vi "Read userEventRef.vi"(8 "error in (no error)":errorcluster, 11 "BoolUserEventStopMechanism In":refnum<class "BoolUETaskChannel.lvclass">) -> (0 "error out":errorcluster, 2 "stopUserEvent":refnum<user-event>, 3 "BoolUserEventStopMechanism Out":refnum<class "BoolUETaskChannel.lvclass">)   [LabVIEW 2023, in "TLC_Daemon.lvlib" / "BoolUETaskChannel.lvclass"]
uses:
  BoolUETaskChannel.lvclass
  BoolUETaskChannel.lvclass/BoolUETaskChannel.ctl
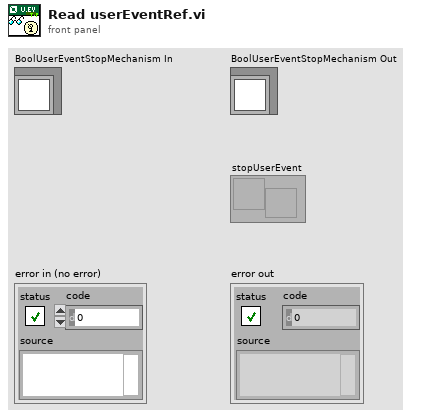
[diagram p1: front panel]
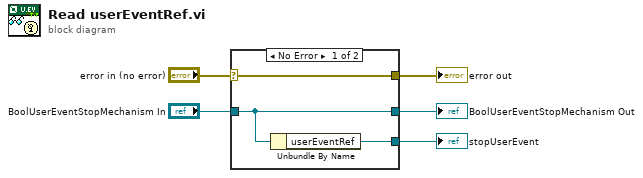
[diagram p0: block diagram]
diagram:
  n1 = case shown="No Error" "error in (no error)" {
    selector: "error in (no error)" -> [w8 w9]
    tunnel: [w8 w9] -> w4
    tunnel: [w7 w10] -> w2
    tunnel: "BoolUserEventStopMechanism In" -> [w7 w10]
    tunnel: [w6 _] -> w1
    frame No Error {
      n2 = Unbundle By Name(w7) -> ("userEventRef"=w6:refnum<user-event>)
    }
    frame Error {
    }
  }
  "error out" <- w4
  "BoolUserEventStopMechanism Out" <- w2
  "stopUserEvent" <- w1
